vi "DrawEllipseDistanceBetweenPoints.vi"(8 "b":dbl, 9 "a":dbl, 10 "t":dbl, 11 "Dt":dbl) -> (1 "(Ds)'":dbl, 3 "Ds":dbl)   [LabVIEW 2017]
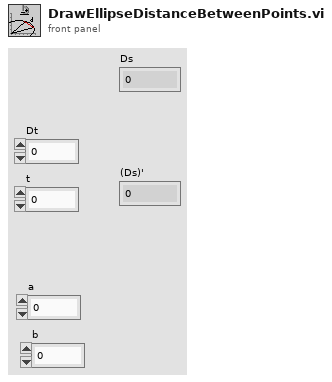
[diagram p1: front panel]
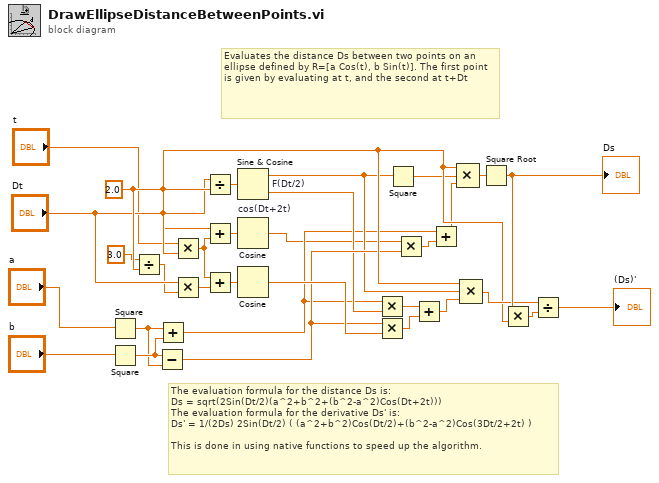
[diagram p0: block diagram]
diagram:
  w28 = 2.0 ("y")
  # "The evaluation formula for the distance Ds is:\nDs = sqrt(2Sin(Dt/2)(a^2+b^2+(b^2-a^2)Cos(Dt+2t)))\nThe evaluation formula for the derivative Ds' is:\nDs' = 1/(2Ds) 2Sin(Dt/2) ( (a^2+b^2)Cos(Dt/2)+(b^2-a^2)Cos(3Dt/2+2t) )\n\nThis is done in using native functions to speed up the algorithm."
  # "Evaluates the distance Ds between two points on an ellipse defined by R=[a Cos(t), b Sin(t)]. The first point is given by evaluating at t, and the second at t+Dt"
  n1 = Square(x="a") -> (x^2=w6:dbl)
  n2 = Square(x="b") -> (x^2=w7:dbl)
  n3 = Divide(x=3.0 ("y"), y=w28) -> (x/y=w15:dbl)
  n4 = Subtract(x=w7, y=w6) -> (x-y=w22:dbl)
  n5 = Add(x=w6, y=w7) -> (x+y=w18:dbl)
  n6 = Multiply(x="t", y=w28) -> (x*y=w14:dbl)
  n7 = Multiply(x="Dt", y=w15) -> (x*y=w16:dbl)
  n8 = Divide(x="Dt", y=w28) -> (x/y=w1:dbl)
  n9 = Add(x="Dt", y=w14) -> (x+y=w2:dbl)
  n10 = Add(x=w14, y=w16) -> (x+y=w13:dbl)
  n11 = Sine & Cosine "F(Dt/2)"(0:w1) -> (1:w19:dbl, 2:w21:dbl)
  n12 = Cosine "cos(Dt+2t)"(x=w2) -> (cos(x)=w11:dbl)
  n13 = Cosine(x=w13) -> (cos(x)=w23:dbl)
  n14 = Multiply(x=w18, y=w21) -> (x*y=w20:dbl)
  n15 = Multiply(x=w22, y=w23) -> (x*y=w24:dbl)
  n16 = Square(x=w19) -> (x^2=w10:dbl)
  n17 = Multiply(x=w11, y=w22) -> (x*y=w8:dbl)
  n18 = Add(x=w20, y=w24) -> (x+y=w17:dbl)
  n19 = Add(x=w18, y=w8) -> (x+y=w9:dbl)
  n20 = Compound Arithmetic op=MULTIPLY(w28, w10, w9) -> (w26:dbl)
  n21 = Compound Arithmetic op=MULTIPLY(w28, w19, w17) -> (w29:dbl)
  n22 = Square Root(x=w26) -> (sqrt(x)=w31:dbl)
  "Ds" <- w31
  n23 = Multiply(x=w31, y=w28) -> (x*y=w27:dbl)
  n24 = Divide(x=w29, y=w27) -> (x/y=→"(Ds)'":dbl)
